vi "SetInit.vi"(6 "Legacy (f)?":bool, 8 "error in (no error)":errorcluster) -> (0 "error out":errorcluster)   [LabVIEW 2011]
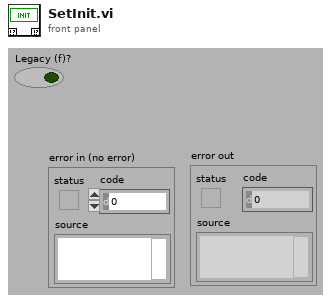
[diagram p1: front panel]
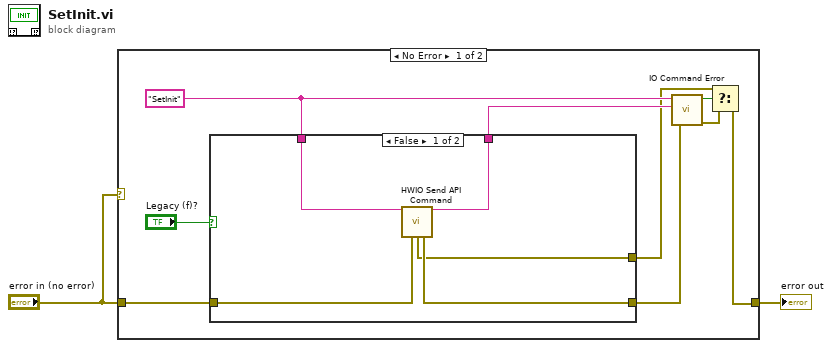
[diagram p0: block diagram]
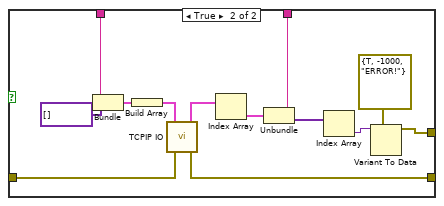
[diagram p2: hidden frame]
diagram:
  n1 = case shown="No Error" "error in (no error)" {
    tunnel: "error in (no error)" -> [w11 w30]
    tunnel: [w6 w30] -> w2
    frame No Error {
      w9 = "SetInit"
      n2 = case shown="False" "Legacy (f)?" {
        tunnel: w11 -> [w16 w28]
        tunnel: [w15 w26] -> w10
        tunnel: w9 -> [w13 w25]
        tunnel: [w14 w21] -> w8
        tunnel: [w12 w17] -> w4
        frame False {
          n3 = call "HWIO Send API Command.vi"("Action"=w13, "error in (no error)"=w16) -> ("Action out"=w14:string, "HWError"=w12:errorcluster, "error out"=w15:errorcluster)  [unwired: 6 in, 5 out]
        }
        frame True {
          n4 = Bundle(w25, variant[] []) -> (w27:cluster{string, variant[]})  [unwired: 1 out]
          n5 = Build Array(w27) -> (w24:cluster{string, variant[]}[])
          n6 = call "TCPIP IO.vi"("error in (no error)"=w28, "Commands"=w24) -> ("error out"=w26:errorcluster, "Responses"=w22:cluster{string, variant[]}[])  [unwired: 1 in, 3 out]
          n7 = Index Array(array=w22) -> (element=w23:cluster{string, variant[]})  [unwired: 1 in]
          n8 = Unbundle(w23) -> (w21:string, w18:variant[])
          n9 = Index Array(array=w18) -> (element=w20:variant)  [unwired: 1 in]
          n10 = Variant To Data(type=errorcluster {"status"=TRUE, "code"=-1000, "source"="ERROR!"} ("error out"), Variant=w20) -> (data=w17:errorcluster)  [unwired: 1 in, 1 out]
        }
      }
      n11 = call "IO Command Error.vi"("error in (no error)"=w10, "Command Returned (\"\")"=w8, "Command Sent (\"\")"=w9) -> ("error out"=w5:errorcluster, "HW ERR?"=w7:bool)  [unwired: 3 out]
      n12 = Select(t=w4, s=w7, f=w5) -> (s? t:f=w6:errorcluster)
    }
    frame Error {
    }
  }
  "error out" <- w2
